vi "get HMI Messages Paths.vi"() -> (2 "PC Messages":path, 3 "PLC Messages":path)   [LabVIEW 2015]
uses:
  Re-use Libraries/Utility/Get App Paths.vi
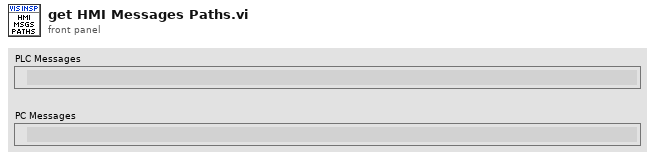
[diagram p1: front panel]
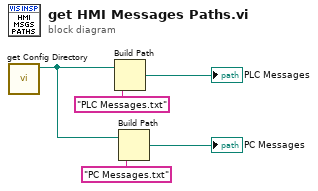
[diagram p0: block diagram]
diagram:
  n1 = call "get Config Directory.vi"() -> ("Config Dir"=w1:path)  [unwired: 11 in]
  n2 = Build Path(base path=w1, name or relative path="PLC Messages.txt") -> (appended path=→"PLC Messages":path)
  n3 = Build Path(base path=w1, name or relative path="PC Messages.txt") -> (appended path=→"PC Messages":path)
